vi "json Query - array path.vi"(8 "error in (no error)":errorcluster, 10 "path":string[](array[string]), 11 "JSON Document in":refnum<class "JSON Document.lvclass">) -> (0 "error out":errorcluster, 1 "type":T1, 2 "found?":bool, 3 "JSON Document out":refnum<class "JSON Document.lvclass">)   [LabVIEW 2016, in "JSON Document.lvclass"]
uses:
  JSON Document.lvclass
  rapidjson wrapper/jsonType.ctl
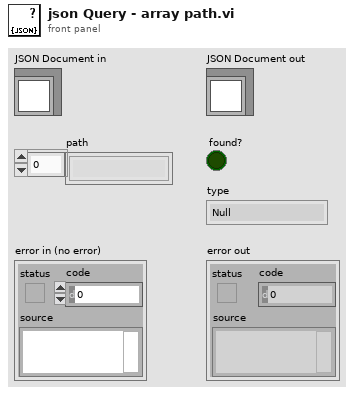
[diagram p1: front panel]
types:
  T1 = typedef "JSON Document.lvclass/jsonType.ctl" = enum16{"Null", "False", "True", "Object", "Array", "String", "Number"}
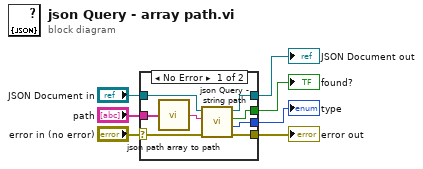
[diagram p0: block diagram]
diagram:
  n1 = case shown="No Error" "error in (no error)" {
    selector: "error in (no error)" -> [w10 w17]
    tunnel: [w11 w17] -> w6
    tunnel: [w14 w16] -> w4
    tunnel: "JSON Document in" -> [w15 w16]
    tunnel: "path" -> [w9 _]
    tunnel: [w13 _] -> w2
    tunnel: [w12 _] -> w1
    frame No Error {
      n2 = call "json path array to path.vi"("path"=w9) -> ("String"=w8:string)
      n3 = call "json Query - string path.vi"("error in (no error)"=w10, "path"=w8, "JSON Document in"=w15) -> ("error out"=w11:errorcluster, "type"=w12:T1, "found?"=w13:bool, "JSON Document out"=w14:refnum<class "JSON Document.lvclass">)  [unwired: 5 in]
    }
    frame Error {
    }
  }
  "error out" <- w6
  "JSON Document out" <- w4
  "type" <- w1
  "found?" <- w2
